vi "myFreqFFTindex.vi"(0 "n_timebase_0":u32, 1 "n_sample_0":u64, 3 "f_fun":u32, 5 "freqs_index":i32, 6 "sweep_mode":u8, 7 "f_freq":i32, 8 "n_timebase_f":u32, 9 "n_sample_f":u64, 10 "fft_index_in":i32[][](array[numeric]), 11 "f_max":i32) -> (2 "fft_index_out":i32[][](array[numeric]))   [LabVIEW 2024]
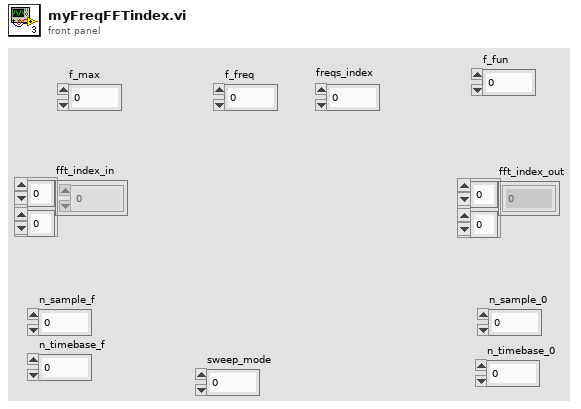
[diagram p1: front panel]
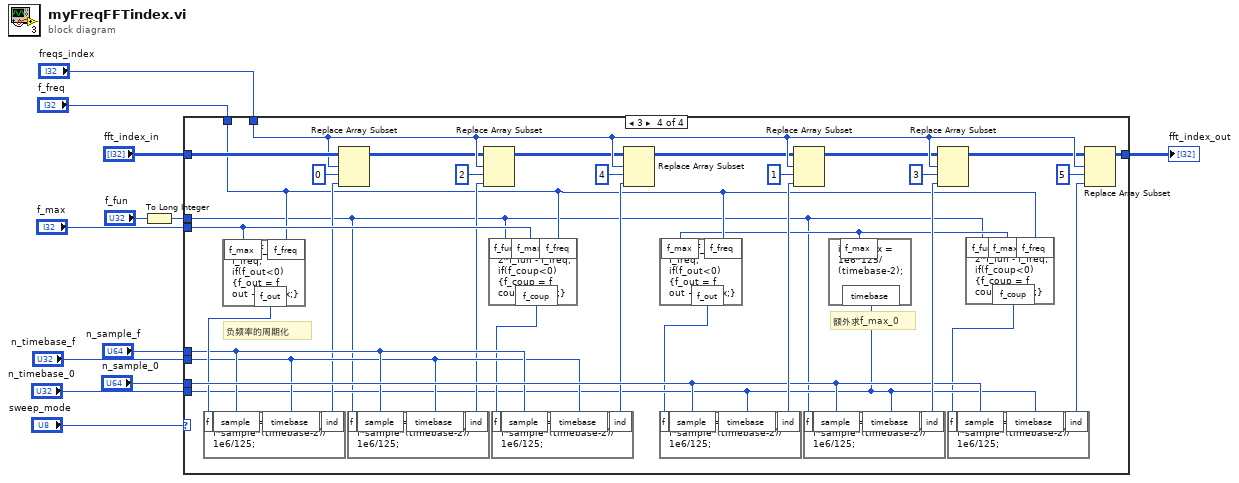
[diagram p0: block diagram]
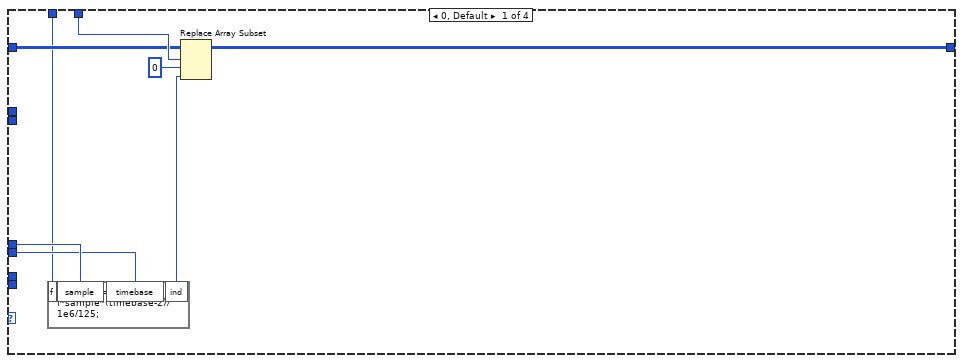
[diagram p2: hidden frame]
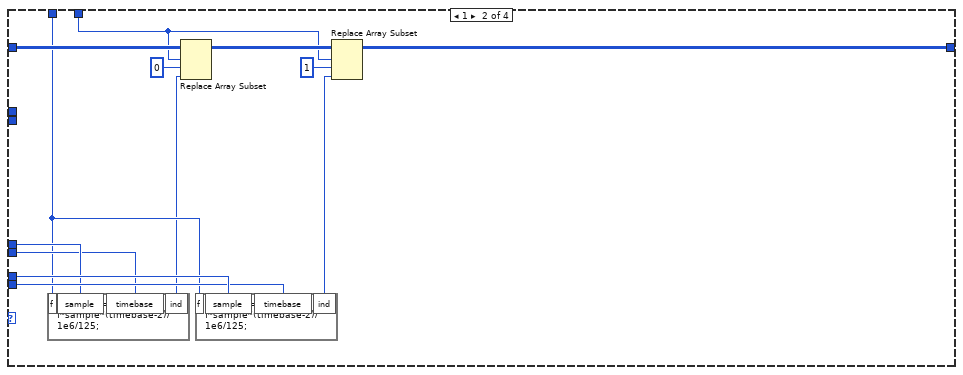
[diagram p3: hidden frame]
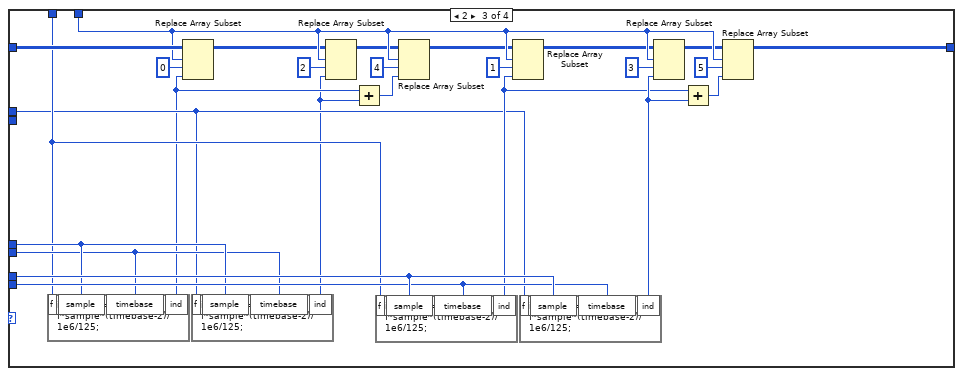
[diagram p4: hidden frame]
diagram:
  n1 = To Long Integer(number="f_fun") -> (32bit integer=w8:i32)
  n2 = case shown="3" "sweep_mode" {
    tunnel: "freqs_index" -> [w20 w28 w50 w83]
    tunnel: "fft_index_in" -> [w19 w32 w58 w88]
    tunnel: [w17 w30 w54 w84] -> w6
    tunnel: w8 -> [_ _ w41 w62]
    tunnel: "f_max" -> [_ _ _ w78]
    tunnel: "f_freq" -> [w14 w22 w42 w64]
    tunnel: "n_sample_0" -> [_ w27 w49 w79]
    tunnel: "n_timebase_0" -> [_ w26 w48 w65]
    tunnel: "n_sample_f" -> [w16 w24 w44 w76]
    tunnel: "n_timebase_f" -> [w15 w23 w43 w75]
    frame 0, Default {
      n3 = formula code="int32 ind = f*sample*(timebase-2)/1e6/125;"("f"=w14, "sample"=w16, "timebase"=w15) -> ("ind"=w13:i32)
      n4 = Replace Array Subset(array=w19, new element=w13, index (row)=w20, index (col)=0 ("索引 (列)")) -> (w17:i32[][])
    }
    frame 1 {
      n5 = formula code="int32 ind = f*sample*(timebase-2)/1e6/125;"("f"=w22, "sample"=w24, "timebase"=w23) -> ("ind"=w21:i32)
      n6 = Replace Array Subset(array=w32, new element=w21, index (row)=w28, index (col)=0 ("索引 (列)")) -> (w31:i32[][])
      n7 = formula code="int32 ind = f*sample*(timebase-2)/1e6/125;"("f"=w22, "sample"=w27, "timebase"=w26) -> ("ind"=w25:i32)
      n8 = Replace Array Subset(array=w31, new element=w25, index (row)=w28, index (col)=1 ("索引 (列)")) -> (w30:i32[][])
    }
    frame 2 {
      n9 = formula code="int32 ind = f*sample*(timebase-2)/1e6/125;"("f"=w42, "sample"=w44, "timebase"=w43) -> ("ind"=w40:i32)
      n10 = Replace Array Subset(array=w58, new element=w40, index (row)=w50, index (col)=0 ("索引 (列)")) -> (w38:i32[][])
      n11 = formula code="int32 ind = f*sample*(timebase-2)/1e6/125;"("f"=w41, "sample"=w44, "timebase"=w43) -> ("ind"=w39:i32)
      n12 = Replace Array Subset(array=w38, new element=w39, index (row)=w50, index (col)=2 ("索引 (列)")) -> (w37:i32[][])
      n13 = Add(x=w40, y=w39) -> (x+y=w55:i32)
      n14 = formula code="int32 ind = f*sample*(timebase-2)/1e6/125;"("f"=w42, "sample"=w49, "timebase"=w48) -> ("ind"=w46:i32)
      n15 = Replace Array Subset(array=w37, new element=w55, index (row)=w50, index (col)=4 ("索引 (列)")) -> (w36:i32[][])
      n16 = Replace Array Subset(array=w36, new element=w46, index (row)=w50, index (col)=1 ("索引 (列)")) -> (w35:i32[][])
      n17 = formula code="int32 ind = f*sample*(timebase-2)/1e6/125;"("f"=w41, "sample"=w49, "timebase"=w48) -> ("ind"=w47:i32)
      n18 = Replace Array Subset(array=w35, new element=w47, index (row)=w50, index (col)=3 ("索引 (列)")) -> (w34:i32[][])
      n19 = Add(x=w46, y=w47) -> (x+y=w45:i32)
      n20 = Replace Array Subset(array=w34, new element=w45, index (row)=w50, index (col)=5 ("索引 (列)")) -> (w54:i32[][])
    }
    frame 3 {
      # "额外求f_max_0"
      # "负频率的周期化"
      n21 = formula code="int32 f_out = f_freq; \nif(f_out<0)\n{f_out = f_out + f_max;}"("f_max"=w78, "f_freq"=w64) -> ("f_out"=w77:i32)
      n22 = formula code="int32 ind = f*sample*(timebase-2)/1e6/125;"("f"=w77, "sample"=w76, "timebase"=w75) -> ("ind"=w74:i32)
      n23 = Replace Array Subset(array=w88, new element=w74, index (row)=w83, index (col)=0 ("索引 (列)")) -> (w70:i32[][])
      n24 = formula code="int32 ind = f*sample*(timebase-2)/1e6/125;"("f"=w62, "sample"=w76, "timebase"=w75) -> ("ind"=w73:i32)
      n25 = Replace Array Subset(array=w70, new element=w73, index (row)=w83, index (col)=2 ("索引 (列)")) -> (w69:i32[][])
      n26 = formula code="int32 f_coup = 2*f_fun - f_freq;\nif(f_coup<0)\n{f_coup = f_coup+f_max;}"("f_fun"=w62, "f_max"=w78, "f_freq"=w64) -> ("f_coup"=w72:i32)
      n27 = formula code="int32 ind = f*sample*(timebase-2)/1e6/125;"("f"=w72, "sample"=w76, "timebase"=w75) -> ("ind"=w71:i32)
      n28 = Replace Array Subset(array=w69, new element=w71, index (row)=w83, index (col)=4 ("索引 (列)")) -> (w68:i32[][])
      n29 = formula code="int32 ind = f*sample*(timebase-2)/1e6/125;"("f"=w62, "sample"=w79, "timebase"=w65) -> ("ind"=w81:i32)
      n30 = formula code="int f_max = 1e6*125/(timebase-2);"("timebase"=w65) -> ("f_max"=w63:i32)
      n31 = formula code="int32 f_out = f_freq; \nif(f_out<0)\n{f_out = f_out + f_max;}"("f_max"=w63, "f_freq"=w64) -> ("f_out"=w60:i32)
      n32 = formula code="int32 ind = f*sample*(timebase-2)/1e6/125;"("f"=w60, "sample"=w79, "timebase"=w65) -> ("ind"=w82:i32)
      n33 = Replace Array Subset(array=w68, new element=w82, index (row)=w83, index (col)=1 ("索引 (列)")) -> (w67:i32[][])
      n34 = Replace Array Subset(array=w67, new element=w81, index (row)=w83, index (col)=3 ("索引 (列)")) -> (w66:i32[][])
      n35 = formula code="int32 f_coup = 2*f_fun - f_freq;\nif(f_coup<0)\n{f_coup = f_coup+f_max;}"("f_fun"=w62, "f_max"=w63, "f_freq"=w64) -> ("f_coup"=w61:i32)
      n36 = formula code="int32 ind = f*sample*(timebase-2)/1e6/125;"("f"=w61, "sample"=w79, "timebase"=w65) -> ("ind"=w80:i32)
      n37 = Replace Array Subset(array=w66, new element=w80, index (row)=w83, index (col)=5 ("索引 (列)")) -> (w84:i32[][])
    }
  }
  "fft_index_out" <- w6
